vi "Get Default Report Path.vi"() -> (2 "Default Report Directory":path, 3 "Default Report Path":path)   [LabVIEW 2020, in "Utilities.lvlib"]
uses:
  Utilities.lvlib
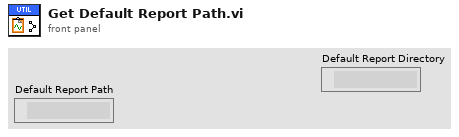
[diagram p1: front panel]
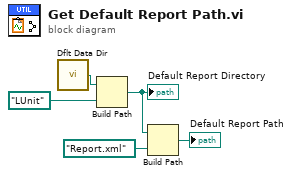
[diagram p0: block diagram]
diagram:
  n1 = call <vilib>:"Dflt Data Dir.vi"() -> ("App:Default Data Directory"=w4:path)
  n2 = Build Path(base path=w4, name or relative path=path "LUnit") -> (appended path=w1:path)
  "Default Report Directory" <- w1
  n3 = Build Path(base path=w1, name or relative path=path "Report.xml") -> (appended path=→"Default Report Path":path)
